vi "Set ROI entry window UI from file-DBL.vi"(8 "error in (no error)":errorcluster, 9 "Keys setup.DBL":T2, 10 "Section name":string, 11 "Refnum in":T1) -> (0 "error out":errorcluster, 3 "Refnum out":T1)   [LabVIEW 2020]
uses:
  Typedefs/Ini file interface (DBL).ctl
  <vilib>/Utility/config.llb/Config Data RefNum.ctl
  User Interface/ROI Entry screen/Globals/gl_ROI Entry UI globals.vi
  <vilib>/Utility/config.llb/NI_LVConfig.lvlib
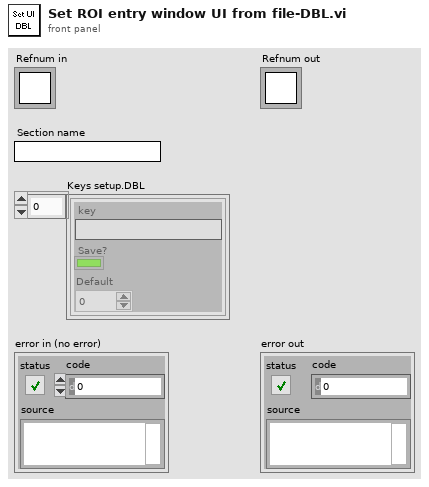
[diagram p1: front panel]
types:
  T1 = typedef "NI_LVConfig.lvlib/Config Data RefNum.ctl" = refnum<k1>
  T2 = typedef "Ini file interface (DBL).ctl" = cluster{"key":string, "Save?":bool, "Default":dbl}[]
  T3 = typedef "ROI entry screen ctrl refs cluster.ctl" = cluster{"Done button":refnum<vi>, "Imaging button":refnum<vi>, "Acquisition button":refnum<vi>, "Scan dwell time per pixel (us)":refnum<vi>, "# of planes":refnum<vi>, "Zoom Ctrl":refnum<vi>, "Equal size":refnum<vi>, "Channel":refnum<vi>, "Image Display":refnum<vi>, "Z-Plane Selector":refnum<vi>, "Number of lines left":refnum<vi>, "Z-stack folder path":refnum<vi>, "POI Density":refnum<vi>, "Arb Plane Entry":refnum<vi>, "Whole Plane":refnum<vi>, "Line Mode":refnum<vi>, "Clear Last":refnum<vi>, "Clear All":refnum<vi>, "Delete Lines":refnum<vi>, "Trial Length (sec)":refnum<vi>, "Palette Type":refnum<vi>, "Intensity slider":refnum<vi>, "# POI":refnum<vi>, "Max Z Proj":refnum<vi>, "Zplane ind":refnum<vi>, "Wavelength (nm)":refnum<vi>, "Number of Trials":refnum<vi>, "Funct stim.trig.enable":refnum<vi>, "Funct stim.trig.delay (s)":refnum<vi>, "Line Mode":refnum<vi>, "Step size (µm)":refnum<vi>, "ROI move mode":refnum<vi>, "Cool-down time (s)":refnum<vi>, "Enable cool-down time":refnum<vi>, "Motor Z ind. (um)":refnum<vi>, "AOL Z ind. (um)":refnum<vi>, "Load Reference Image":refnum<vi>, "Rel.  Res.":refnum<vi>, "ROI LIST":refnum<vi>, "Show All":refnum<vi>, "ROI Type":refnum<vi>, "Start Plane":refnum<vi>, "Stop Plane":refnum<vi>, "Offset ROI":refnum<vi>, "Tab Control":refnum<vi>, "Laser Power(%)":refnum<vi>, "Cycle rate":refnum<vi>, "FOV (Ind.)":refnum<vi>, "Frame Size (Ind.)":refnum<vi>, "Resolution (Ind.)":refnum<vi>, "Pixel Density (Ind)":refnum<vi>, "Laser Power (Ind.)":refnum<vi>, "Dwell Time (Ind.)":refnum<vi>, "Adj MC":refnum<vi>}
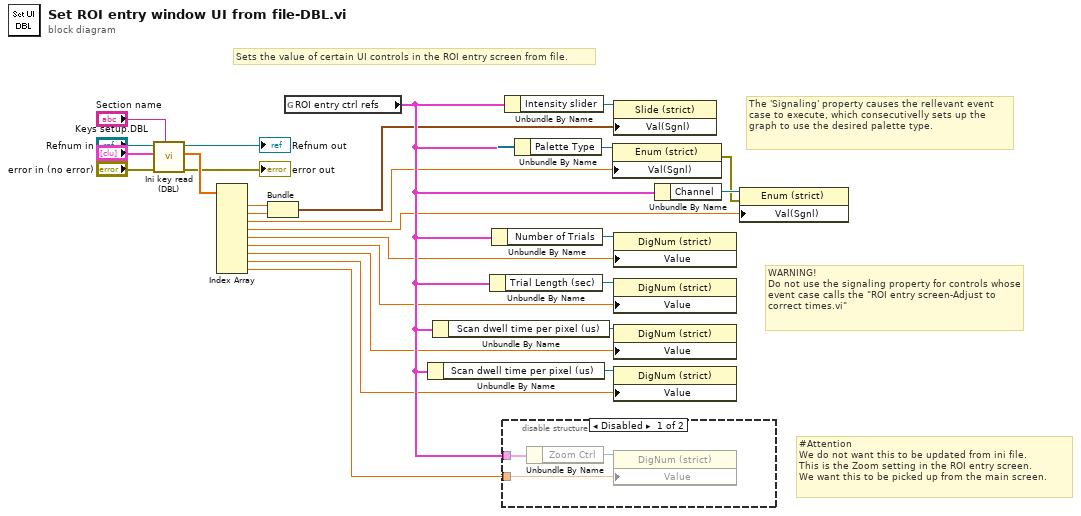
[diagram p0: block diagram]
diagram:
  # "#Attention\nWe do not want this to be updated from ini file.\nThis is the Zoom setting in the ROI entry screen.\nWe want this to be picked up from the main screen."
  # "WARNING!\nDo not use the signaling property for controls whose event case calls the \"ROI entry screen-Adjust to correct times.vi\""
  # "The 'Signaling' property causes the rellevant event case to execute, which consecutivelly sets up the graph to use the desired palette type."
  # "Sets the value of certain UI controls in the ROI entry screen from file."
  n1 = call "Ini key read (DBL).vi"("Section name"="Section name", "error in (no error)"="error in (no error)", "Parameter names & setup"="Keys setup.DBL", "Ini file refnum in"="Refnum in") -> ("error out"=→"error out":errorcluster, "Value read/used"=w24:dbl[], "Ini file refnum out"=→"Refnum out":T1)  [unwired: 5 in]
  n2 = Index Array(array=w24) -> (element #1=w11:dbl, element #2=w10:dbl, element #3=w2:dbl, element #4=w8:dbl, element #5=w7:dbl, element #6=w6:dbl, element #7=w5:dbl, element #8=w4:dbl, element #9=w3:dbl)  [unwired: 9 in]
  n3 = Bundle("value"=w11, "value"=w10) -> (w9:cluster{"value":dbl, "value":dbl})  [unwired: 1 in]
  n4 = global read "gl_ROI Entry UI globals.vi" "ROI entry ctrl refs"() -> (w12:T3)
  n5 = Unbundle By Name(w12) -> ("Scan dwell time per pixel (us)"=w13:refnum<vi>)
  n6 = Unbundle By Name(w12) -> ("Scan dwell time per pixel (us)"=w14:refnum<vi>)
  n7 = Unbundle By Name(w12) -> ("Trial Length (sec)"=w17:refnum<vi>)
  n8 = Unbundle By Name(w12) -> ("Number of Trials"=w16:refnum<vi>)
  n9 = disable-structure shown="Disabled" {
    disable-tunnel: w12 -> [w28 _]
    disable-tunnel: w3 -> [w27 _]
    frame Disabled {
      n10 = Unbundle By Name(w28) -> ("Zoom Ctrl"=w29:refnum<vi>)
      n11 = property class="DigNum (strict)"(reference=w29, "Value"=w27) -> ()  [unwired: 1 in, 2 out]
    }
    frame Enabled {
    }
  }
  n12 = Unbundle By Name(w12) -> ("Intensity slider"=w15:refnum<vi>)
  n13 = Unbundle By Name(w12) -> ("Palette Type"=w19:refnum<vi>)
  n14 = property class="Enum (strict)"(reference=w19, "Val(Sgnl)"=w2) -> (error out=w1:errorcluster)  [unwired: 1 in, 1 out]
  n15 = property class="Slide (strict)"(reference=w15, "Val(Sgnl)"=w9) -> ()  [unwired: 1 in, 2 out]
  n16 = property class="DigNum (strict)"(reference=w16, "Value"=w7) -> ()  [unwired: 1 in, 2 out]
  n17 = property class="DigNum (strict)"(reference=w17, "Value"=w6) -> ()  [unwired: 1 in, 2 out]
  n18 = property class="DigNum (strict)"(reference=w14, "Value"=w5) -> ()  [unwired: 1 in, 2 out]
  n19 = property class="DigNum (strict)"(reference=w13, "Value"=w4) -> ()  [unwired: 1 in, 2 out]
  n20 = Unbundle By Name(w12) -> ("Channel"=w18:refnum<vi>)
  n21 = property class="Enum (strict)"(reference=w18, error in=w1, "Val(Sgnl)"=w8) -> ()  [unwired: 2 out]
